vi "refractiveIndex_infoIMPORT.vi"() -> ()   [LabVIEW 2014]
uses:
  <vilib>/Utility/file.llb/Read From Spreadsheet File (DBL).vi
  <vilib>/Utility/file.llb/Write To Spreadsheet File (DBL).vi
panel:
  out "deleted portion":dbl[][](array[numeric])
  out "index of element":i32
  out "transposed array 2":dbl[][](array[numeric])
  out "transposed array":dbl[][](array[numeric])
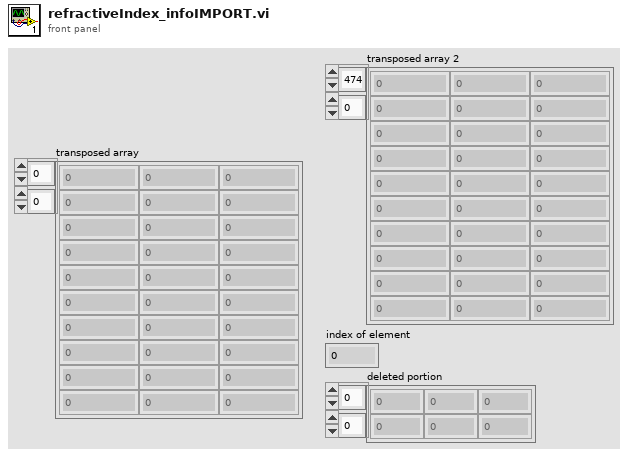
[diagram p1: front panel]
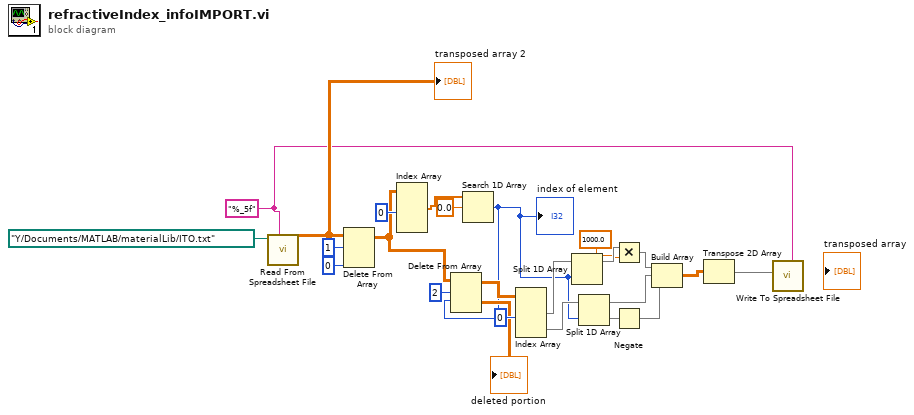
[diagram p0: block diagram]
diagram:
  w1 = "%_5f" ("format (%.3f)")
  n1 = call-poly <vilib>:"Read From Spreadsheet File.vi"("format (%.3f)"=w1, "file path (dialog if empty)"=path "Y:/Documents/MATLAB/materialLib/ITO.txt") -> ("all rows"=w10:dbl[][])  [unwired: 5 in, 4 out]
  "transposed array 2" <- w10
  n2 = Delete From Array(array=w10, length=1, index (row)=0) -> (array with subset deleted=w18:dbl[][])  [unwired: 1 in, 1 out]
  n3 = Index Array(array=w18, index (col) #1=0 ("disabled index (col)")) -> (element #1=w19:dbl[])  [unwired: 3 in, 1 out]
  n4 = Search 1D Array(1D array=w19, element=0.0) -> (index of element=w8:i32)  [unwired: 1 in]
  "index of element" <- w8
  n5 = Delete From Array(array=w18, length=2, index (row)=w8) -> (deleted portion=→"deleted portion":dbl[][], array with subset deleted=w16:dbl[][])  [unwired: 1 in]
  n6 = Index Array(array=w16, index (col) #1=0 ("disabled index (col)")) -> (element #1=w14:dbl[], element #2=w13:dbl[])  [unwired: 3 in]
  n7 = Split 1D Array(array=w14, index=w8) -> (first subarray=w7:dbl[])  [unwired: 1 out]
  n8 = Split 1D Array(array=w13, index=w8) -> (first subarray=w12:dbl[], second subarray=w4:dbl[])
  n9 = Multiply(x=w7, y=1000.0) -> (x*y=w5:dbl[])
  n10 = Negate(x=w4) -> (-x=w3:dbl[])
  n11 = Build Array(w5, w12, w3) -> (w11:dbl[][])
  n12 = Transpose 2D Array(2D array=w11) -> (transposed array=w2:dbl[][])
  n13 = call-poly <vilib>:"Write To Spreadsheet File.vi"("format (%.3f)"=w1, "2D data"=w2) -> ()  [unwired: 6 in, 1 out]
